vi "lib Time String to Time Stamp.vi"(7 "Default":timestamp, 8 "error in (no error)":errorcluster, 10 "Format":T1, 11 "Array of time strings":string[](array[string])) -> (0 "error out":errorcluster, 3 "Array":timestamp[](array[timestamp]) format="%<%H:%M:%S%3u\n%x>T")   [LabVIEW 2024]
doc: "Convert string time specification in the format \"2010-04-28 09:39:06\" to LabVIEW timestamp type in LabVIEW time Epoch."
uses:
  Time/lib enum String Time Format.ctl
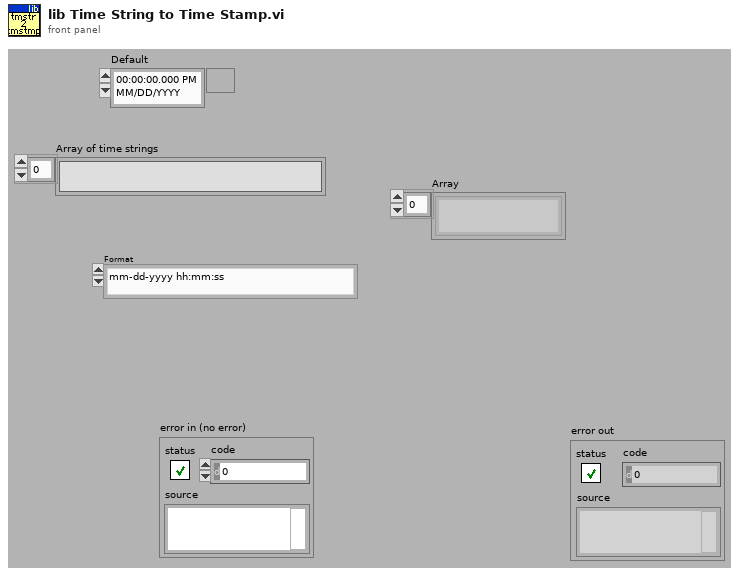
[diagram p1: front panel]
types:
  T1 = typedef "lib enum String Time Format.ctl" = enum16{"mm-dd-yyyy hh:mm:ss", "yy-doy-hh:mm:ss", "m/d/y hh:mm:ss", "yyyy-mm-dd hh:mm:ss", "yy/doy-hh:mm:ss", "mm-dd-yyyy", "hh:mm:ss"}
  T2 = typedef "LVDateTimeRec.ctl" = cluster{"fractional second":dbl, "second":i32, "minute":i32, "hour":i32, "day of month":i32, "month":i32, "year":i32, "day of week":i32, "day of year":i32, "DST":i32}
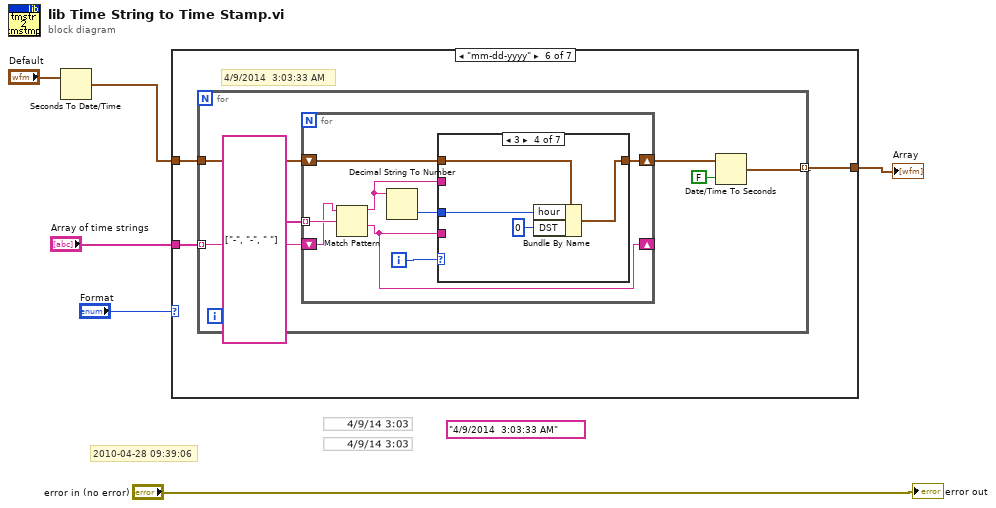
[diagram p0: block diagram]
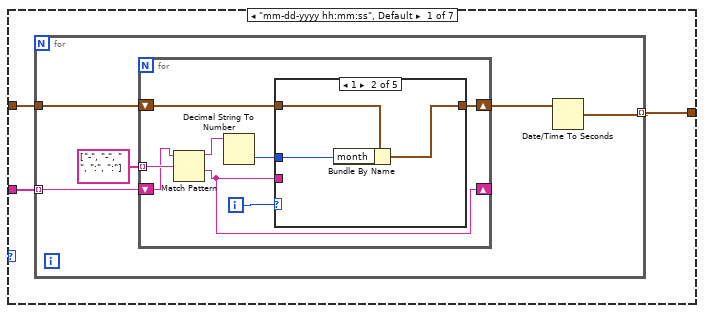
[diagram p2: hidden frame]
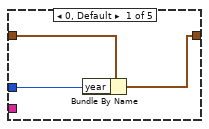
[diagram p3: hidden frame]
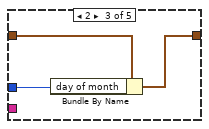
[diagram p4: hidden frame]
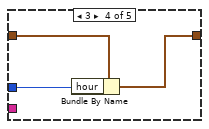
[diagram p5: hidden frame]
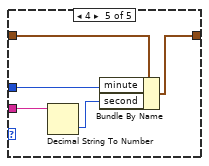
[diagram p6: hidden frame]
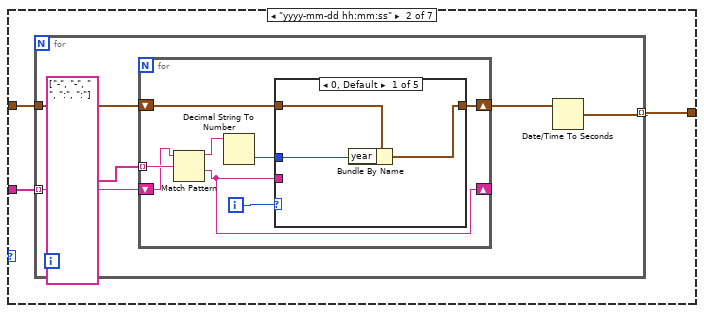
[diagram p7: hidden frame]
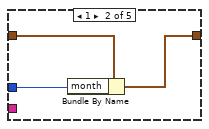
[diagram p8: hidden frame]
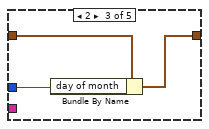
[diagram p9: hidden frame]
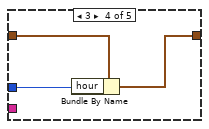
[diagram p10: hidden frame]
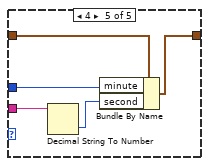
[diagram p11: hidden frame]
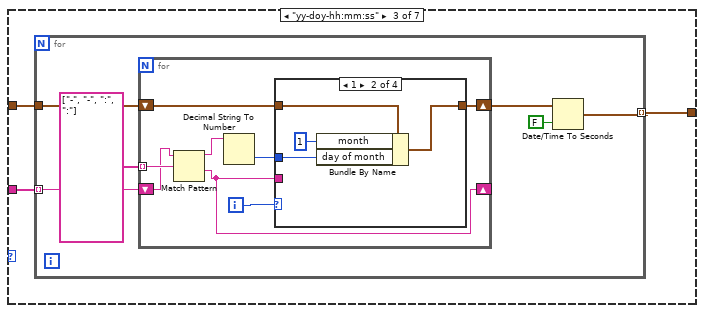
[diagram p12: hidden frame]
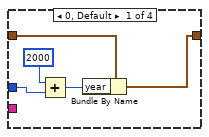
[diagram p13: hidden frame]
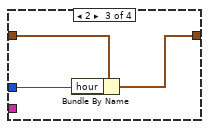
[diagram p14: hidden frame]
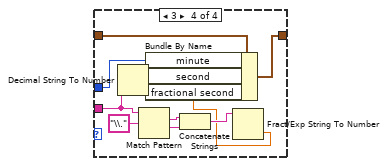
[diagram p15: hidden frame]
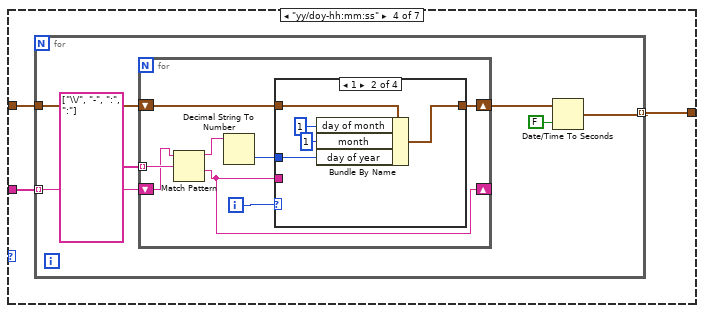
[diagram p16: hidden frame]
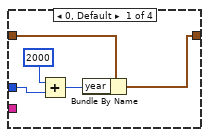
[diagram p17: hidden frame]
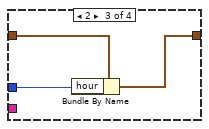
[diagram p18: hidden frame]
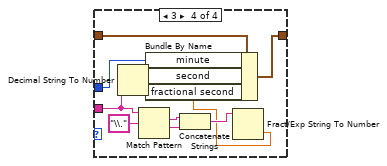
[diagram p19: hidden frame]
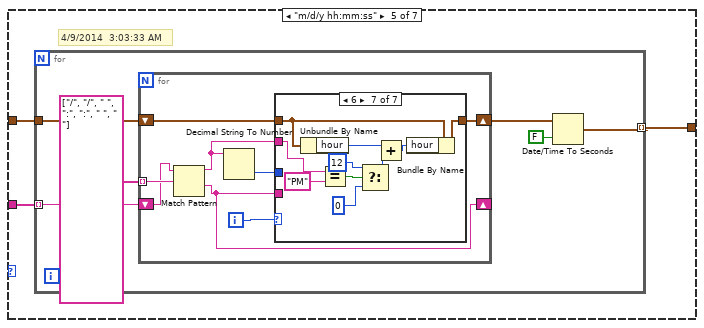
[diagram p20: hidden frame]
diagram:
  (unwired) "4/9/2014  3:03:33 AM"
  # "2010-04-28 09:39:06"
  n1 = Seconds To Date/Time(time stamp (now)="Default") -> (date time rec=w1:T2)  [unwired: 1 in]
  n2 = case shown="\"mm-dd-yyyy\"" "Format" {
    tunnel: w1 -> [w9 w42 w75 w114 w154 w205 w256]
    tunnel: [w8 w41 w74 w113 w153 w204 w255] -> w6
    tunnel: "Array of time strings" -> [w7 w40 w73 w112 w152 w203 w254]
    frame "mm-dd-yyyy hh:mm:ss", Default {
      n3 = for {
        tunnel: w9 -> [w13]
        tunnel: [w11] -> w8 mode=indexing
        tunnel: w7 -> [w10] mode=indexing
        n4 = for {
          tunnel: string[] ["-", "-", " ", ":", ":"] -> [w22] mode=indexing
          shift-right: [w15] -> _
          shift-left: w10 -> [w16]
          shift-right: [w17] -> w12
          shift-left: w13 -> [w18]
          i -> [w21]
          n5 = Match Pattern(string=w16, regular expression=w22) -> (before substring=w20:string, after substring=w15:string)  [unwired: 1 in, 2 out]
          n6 = Decimal String To Number(string=w20) -> (number=w19:i32)  [unwired: 2 in, 1 out]
          n7 = case shown="1" w21 {
            tunnel: w19 -> [w24 w27 w30 w33 w38]
            tunnel: w18 -> [w25 w28 w31 w34 w39]
            tunnel: [w23 w26 w29 w32 w37] -> w17
            tunnel: w15 -> [_ _ _ _ w36]
            frame 0, Default {
              n8 = Bundle By Name(cluster=w25, "year"=w24) -> (w23:T2)
            }
            frame 1 {
              n9 = Bundle By Name(cluster=w28, "month"=w27) -> (w26:T2)
            }
            frame 2 {
              n10 = Bundle By Name(cluster=w31, "day of month"=w30) -> (w29:T2)
            }
            frame 3 {
              n11 = Bundle By Name(cluster=w34, "hour"=w33) -> (w32:T2)
            }
            frame 4 {
              n12 = Decimal String To Number(string=w36) -> (number=w35:i32)  [unwired: 2 in, 1 out]
              n13 = Bundle By Name(cluster=w39, "minute"=w38, "second"=w35) -> (w37:T2)
            }
          }
        }
        n14 = Date/Time To Seconds(2:w12) -> (0:w11:timestamp)  [unwired: 1 in]
      }
    }
    frame "yyyy-mm-dd hh:mm:ss" {
      n15 = for {
        tunnel: w42 -> [w46]
        tunnel: [w44] -> w41 mode=indexing
        tunnel: w40 -> [w43] mode=indexing
        n16 = for {
          tunnel: string[] ["-", "-", " ", ":", ":"] -> [w55] mode=indexing
          shift-right: [w48] -> _
          shift-left: w43 -> [w49]
          shift-right: [w50] -> w45
          shift-left: w46 -> [w51]
          i -> [w54]
          n17 = Match Pattern(string=w49, regular expression=w55) -> (before substring=w53:string, after substring=w48:string)  [unwired: 1 in, 2 out]
          n18 = Decimal String To Number(string=w53) -> (number=w52:i32)  [unwired: 2 in, 1 out]
          n19 = case shown="0, Default" w54 {
            tunnel: w52 -> [w57 w60 w63 w66 w71]
            tunnel: w51 -> [w58 w61 w64 w67 w72]
            tunnel: [w56 w59 w62 w65 w70] -> w50
            tunnel: w48 -> [_ _ _ _ w69]
            frame 0, Default {
              n20 = Bundle By Name(cluster=w58, "year"=w57) -> (w56:T2)
            }
            frame 1 {
              n21 = Bundle By Name(cluster=w61, "month"=w60) -> (w59:T2)
            }
            frame 2 {
              n22 = Bundle By Name(cluster=w64, "day of month"=w63) -> (w62:T2)
            }
            frame 3 {
              n23 = Bundle By Name(cluster=w67, "hour"=w66) -> (w65:T2)
            }
            frame 4 {
              n24 = Decimal String To Number(string=w69) -> (number=w68:i32)  [unwired: 2 in, 1 out]
              n25 = Bundle By Name(cluster=w72, "minute"=w71, "second"=w68) -> (w70:T2)
            }
          }
        }
        n26 = Date/Time To Seconds(2:w45) -> (0:w44:timestamp)  [unwired: 1 in]
      }
    }
    frame "yy-doy-hh:mm:ss" {
      n27 = for {
        tunnel: w75 -> [w80]
        tunnel: [w78] -> w74 mode=indexing
        tunnel: w73 -> [w77] mode=indexing
        n28 = for {
          tunnel: string[] ["-", "-", ":", ":"] -> [w89] mode=indexing
          shift-right: [w82] -> _
          shift-left: w77 -> [w83]
          shift-right: [w84] -> w79
          shift-left: w80 -> [w85]
          i -> [w88]
          n29 = Match Pattern(string=w83, regular expression=w89) -> (before substring=w87:string, after substring=w82:string)  [unwired: 1 in, 2 out]
          n30 = Decimal String To Number(string=w87) -> (number=w86:i32)  [unwired: 2 in, 1 out]
          n31 = case shown="1" w88 {
            tunnel: w86 -> [w93 w97 w100 w110]
            tunnel: w85 -> [w94 w98 w101 w111]
            tunnel: [w92 w96 w99 w109] -> w84
            tunnel: w82 -> [_ _ _ w107]
            frame 0, Default {
              n32 = Add(x=2000, y=w93) -> (x+y=w91:i32)
              n33 = Bundle By Name(cluster=w94, "year"=w91) -> (w92:T2)
            }
            frame 1 {
              n34 = Bundle By Name(cluster=w98, "month"=1, "day of month"=w97) -> (w96:T2)
            }
            frame 2 {
              n35 = Bundle By Name(cluster=w101, "hour"=w100) -> (w99:T2)
            }
            frame 3 {
              n36 = Decimal String To Number(string=w107) -> (number=w108:i32)  [unwired: 2 in, 1 out]
              n37 = Match Pattern(string=w107, regular expression="\\.") -> (match substring=w104:string, after substring=w105:string)  [unwired: 1 in, 2 out]
              n38 = Concatenate Strings(w104, w105) -> (w103:string)
              n39 = Fract/Exp String To Number(string=w103) -> (number=w102:dbl)  [unwired: 3 in, 1 out]
              n40 = Bundle By Name(cluster=w111, "minute"=w110, "second"=w108, "fractional second"=w102) -> (w109:T2)
            }
          }
        }
        n41 = Date/Time To Seconds(1:FALSE ("is UTC (F)"), 2:w79) -> (0:w78:timestamp)
      }
    }
    frame "yy/doy-hh:mm:ss" {
      n42 = for {
        tunnel: w114 -> [w119]
        tunnel: [w117] -> w113 mode=indexing
        tunnel: w112 -> [w116] mode=indexing
        n43 = for {
          tunnel: string[] ["\\/", "-", ":", ":"] -> [w128] mode=indexing
          shift-right: [w121] -> _
          shift-left: w116 -> [w122]
          shift-right: [w123] -> w118
          shift-left: w119 -> [w124]
          i -> [w127]
          n44 = Match Pattern(string=w122, regular expression=w128) -> (before substring=w126:string, after substring=w121:string)  [unwired: 1 in, 2 out]
          n45 = Decimal String To Number(string=w126) -> (number=w125:i32)  [unwired: 2 in, 1 out]
          n46 = case shown="1" w127 {
            tunnel: w125 -> [w132 w137 w140 w150]
            tunnel: w124 -> [w133 w138 w141 w151]
            tunnel: [w131 w136 w139 w149] -> w123
            tunnel: w121 -> [_ _ _ w147]
            frame 0, Default {
              n47 = Add(x=2000, y=w132) -> (x+y=w130:i32)
              n48 = Bundle By Name(cluster=w133, "year"=w130) -> (w131:T2)
            }
            frame 1 {
              n49 = Bundle By Name(cluster=w138, "day of month"=1, "month"=1, "day of year"=w137) -> (w136:T2)
            }
            frame 2 {
              n50 = Bundle By Name(cluster=w141, "hour"=w140) -> (w139:T2)
            }
            frame 3 {
              n51 = Decimal String To Number(string=w147) -> (number=w148:i32)  [unwired: 2 in, 1 out]
              n52 = Match Pattern(string=w147, regular expression="\\.") -> (match substring=w144:string, after substring=w145:string)  [unwired: 1 in, 2 out]
              n53 = Concatenate Strings(w144, w145) -> (w143:string)
              n54 = Fract/Exp String To Number(string=w143) -> (number=w142:dbl)  [unwired: 3 in, 1 out]
              n55 = Bundle By Name(cluster=w151, "minute"=w150, "second"=w148, "fractional second"=w142) -> (w149:T2)
            }
          }
        }
        n56 = Date/Time To Seconds(1:FALSE ("is UTC (F)"), 2:w118) -> (0:w117:timestamp)
      }
    }
    frame "m/d/y hh:mm:ss" {
      # "4/9/2014  3:03:33 AM"
      n57 = for {
        tunnel: w154 -> [w159]
        tunnel: [w157] -> w153 mode=indexing
        tunnel: w152 -> [w156] mode=indexing
        n58 = for {
          tunnel: string[] ["/", "/", " ", ":", ":", " ", " "] -> [w168] mode=indexing
          shift-right: [w162] -> _
          shift-left: w156 -> [w163]
          shift-right: [w164] -> w158
          shift-left: w159 -> [w165]
          i -> [w167]
          n59 = Match Pattern(string=w163, regular expression=w168) -> (before substring=w161:string, after substring=w162:string)  [unwired: 1 in, 2 out]
          n60 = Decimal String To Number(string=w161) -> (number=w166:i32)  [unwired: 2 in, 1 out]
          n61 = case shown="6" w167 {
            tunnel: w166 -> [w169 w173 w176 w185 w188 w191 _]
            tunnel: w165 -> [w171 w174 w182 w186 w189 w192 w201]
            tunnel: [w170 w172 w181 w184 w187 w190 w202] -> w164
            tunnel: w162 -> [_ _ _ _ _ _ _]
            tunnel: w161 -> [_ _ _ _ _ _ w200]
            frame 0, Default {
              n62 = Bundle By Name(cluster=w171, "month"=w169) -> (w170:T2)
            }
            frame 1 {
              n63 = Bundle By Name(cluster=w174, "day of month"=w173) -> (w172:T2)
            }
            frame 2 {
              n64 = Add(x=2000, y=w176) -> (x+y=w177:i32)
              n65 = Less?(x=w176, y=100) -> (x < y?=w178:bool)
              n66 = Select(t=w177, s=w178, f=w176) -> (s? t:f=w175:i32)
              n67 = Bundle By Name(cluster=w182, "year"=w175) -> (w181:T2)
            }
            frame 3 {
              n68 = Bundle By Name(cluster=w186, "hour"=w185, "DST"=1) -> (w184:T2)
            }
            frame 4 {
              n69 = Bundle By Name(cluster=w189, "minute"=w188) -> (w187:T2)
            }
            frame 5 {
              n70 = Bundle By Name(cluster=w192, "second"=w191) -> (w190:T2)
            }
            frame 6 {
              n71 = Unbundle By Name(w201) -> ("hour"=w195:i32)
              n72 = Equal?(x=w200, y="PM") -> (x = y?=w198:bool)
              n73 = Select(t=12, s=w198, f=0) -> (s? t:f=w194:i32)
              n74 = Add(x=w195, y=w194) -> (x+y=w193:i32)
              n75 = Bundle By Name(cluster=w201, "hour"=w193) -> (w202:T2)
            }
          }
        }
        n76 = Date/Time To Seconds(1:FALSE ("is UTC (F)"), 2:w158) -> (0:w157:timestamp)
      }
    }
    frame "mm-dd-yyyy" {
      # "4/9/2014  3:03:33 AM"
      n77 = for {
        tunnel: w205 -> [w210]
        tunnel: [w208] -> w204 mode=indexing
        tunnel: w203 -> [w207] mode=indexing
        n78 = for {
          tunnel: string[] ["-", "-", " "] -> [w219] mode=indexing
          shift-right: [w213] -> _
          shift-left: w207 -> [w214]
          shift-right: [w215] -> w209
          shift-left: w210 -> [w216]
          i -> [w218]
          n79 = Match Pattern(string=w214, regular expression=w219) -> (before substring=w212:string, after substring=w213:string)  [unwired: 1 in, 2 out]
          n80 = Decimal String To Number(string=w212) -> (number=w217:i32)  [unwired: 2 in, 1 out]
          n81 = case shown="3" w218 {
            tunnel: w217 -> [w220 w224 w227 w236 w239 w242 _]
            tunnel: w216 -> [w222 w225 w233 w237 w240 w243 w252]
            tunnel: [w221 w223 w232 w235 w238 w241 w253] -> w215
            tunnel: w213 -> [_ _ _ _ _ _ _]
            tunnel: w212 -> [_ _ _ _ _ _ w251]
            frame 0, Default {
              n82 = Bundle By Name(cluster=w222, "month"=w220) -> (w221:T2)
            }
            frame 1 {
              n83 = Bundle By Name(cluster=w225, "day of month"=w224) -> (w223:T2)
            }
            frame 2 {
              n84 = Add(x=2000, y=w227) -> (x+y=w228:i32)
              n85 = Less?(x=w227, y=100) -> (x < y?=w229:bool)
              n86 = Select(t=w228, s=w229, f=w227) -> (s? t:f=w226:i32)
              n87 = Bundle By Name(cluster=w233, "year"=w226) -> (w232:T2)
            }
            frame 3 {
              n88 = Bundle By Name(cluster=w237, "hour"=w236, "DST"=0) -> (w235:T2)
            }
            frame 4 {
              n89 = Bundle By Name(cluster=w240, "minute"=w239) -> (w238:T2)
            }
            frame 5 {
              n90 = Bundle By Name(cluster=w243, "second"=w242) -> (w241:T2)
            }
            frame 6 {
              n91 = Unbundle By Name(w252) -> ("hour"=w246:i32)
              n92 = Equal?(x=w251, y="PM") -> (x = y?=w249:bool)
              n93 = Select(t=12, s=w249, f=0) -> (s? t:f=w245:i32)
              n94 = Add(x=w246, y=w245) -> (x+y=w244:i32)
              n95 = Bundle By Name(cluster=w252, "hour"=w244) -> (w253:T2)
            }
          }
        }
        n96 = Date/Time To Seconds(1:FALSE ("is UTC (F)"), 2:w209) -> (0:w208:timestamp)
      }
    }
    frame "hh:mm:ss" {
      # "4/9/2014  3:03:33 AM"
      n97 = for {
        tunnel: w256 -> [w261]
        tunnel: [w259] -> w255 mode=indexing
        tunnel: w254 -> [w258] mode=indexing
        n98 = for {
          tunnel: string[] [":", ":", " "] -> [w270] mode=indexing
          shift-right: [w264] -> _
          shift-left: w258 -> [w265]
          shift-right: [w266] -> w260
          shift-left: w261 -> [w267]
          i -> [w269]
          n99 = Match Pattern(string=w265, regular expression=w270) -> (before substring=w263:string, after substring=w264:string)  [unwired: 1 in, 2 out]
          n100 = Decimal String To Number(string=w263) -> (number=w268:i32)  [unwired: 2 in, 1 out]
          n101 = case shown="1" w269 {
            tunnel: w268 -> [w272 w276 w279]
            tunnel: w267 -> [w274 w277 w280]
            tunnel: [w273 w275 w278] -> w266
            tunnel: w264 -> [_ _ _]
            tunnel: w263 -> [_ _ _]
            frame 0, Default {
              n102 = Bundle By Name(cluster=w274, "hour"=w272, "DST"=0) -> (w273:T2)
            }
            frame 1 {
              n103 = Bundle By Name(cluster=w277, "minute"=w276) -> (w275:T2)
            }
            frame 2 {
              n104 = Bundle By Name(cluster=w280, "second"=w279) -> (w278:T2)
            }
          }
        }
        n105 = Date/Time To Seconds(1:FALSE ("is UTC (F)"), 2:w260) -> (0:w259:timestamp)
      }
    }
  }
  "Array" <- w6
  "error out" <- "error in (no error)"
